vi "Construct.vi"(8 "Error in (no error)":errorcluster, 10 "Supress":bool=TRUE, 11 "LogFilterSupress in":refnum<class "LogFilterSupress.lvclass">) -> (0 "Error out":errorcluster, 3 "LogFilterSupress out":refnum<class "LogFilterSupress.lvclass">)   [LabVIEW 2011, in "LogFilterSupress.lvclass"]
uses:
  LogFilterSupress.lvclass
  LogFilterSupress.lvclass/LogFilterSupress.ctl
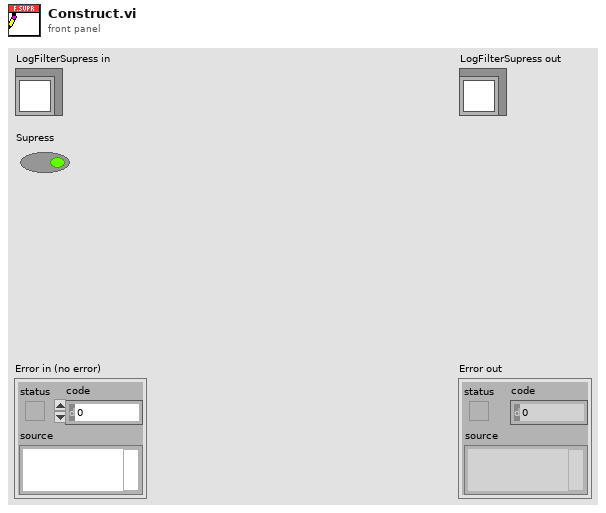
[diagram p1: front panel]
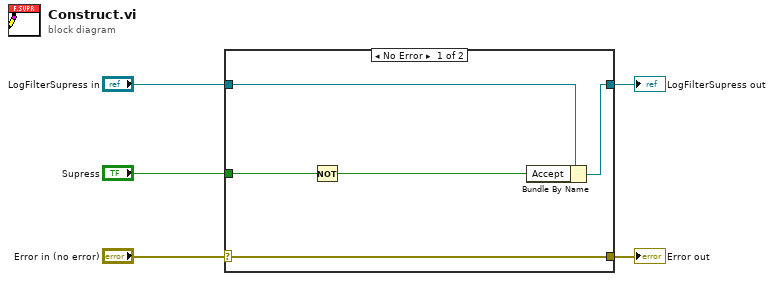
[diagram p0: block diagram]
diagram:
  n1 = case shown="No Error" "Error in (no error)" {
    selector: "Error in (no error)" -> [w10 w11]
    tunnel: [w10 w11] -> w4
    tunnel: [w8 w12] -> w2
    tunnel: "LogFilterSupress in" -> [w9 w12]
    tunnel: "Supress" -> [w7 _]
    frame No Error {
      n2 = Not(x=w7) -> (.not. x?=w6:bool)
      n3 = Bundle By Name(cluster=w9, "Accept"=w6) -> (w8:refnum<class "LogFilterSupress.lvclass">)
    }
    frame Error {
    }
  }
  "Error out" <- w4
  "LogFilterSupress out" <- w2
